vi "Get Text Label Decs from VI__ogtk.vi"(8 "error in (no error)":errorcluster, 11 "VI Refnum":refnum<vi>) -> (0 "error out":errorcluster, 2 "FP Floating Text Labels":refnum<vi>[](array[refnum]), 3 "dup VI Refnum":refnum<vi>)   [LabVIEW 2016]
doc: "Returns references to the free labels (floating text) on a VI's Front Panel."
panel:
  # "Get Text Label Decs from VI.vi\n\nReturns references to the free labels (floating text) on a VI's Front Panel.\n\nPlease visit http://www.OpenG.org to learn about the\nOpen Source LabVIEW software movement.\n\nNOTICE -- YOU MUST LEAVE THIS NOTICE IN PLACE.  PER THE TERMS OF THE LICENSE BELOW, YOU MAY SUBLICENSE THIS SOFTWARE \nIN ANY WAY THAT DOES NOT CONFLICT WITH THIS LICENSE.\n\n### BSD License (http://www.opensource.org/licenses/bsd-license.php) Begin ###\n \nCopyright (c) 2002, Jean-Pierre Drolet <drolet_jp@hotmail.com>\nCopyright (c) 2002, Jim Kring <jim@jimkring.com>\n\nAll rights reserved.\n\nRedistribution and use in source and binary forms, with or without modification, are permitted provided that the following conditions are met:\n\n    * Redistributions of source code must retain the above copyright notice, this list of conditions and the following disclaimer.\n    * Redistributions in binary form must reproduce the above copyright notice, this list of conditions and the following disclaimer in the \n       documentation and/or other materials provided with the distribution.\n    * Neither the name of SciWare, James Kring, Inc., nor the names of its contributors may be used to endorse or promote products derived \n       from this software without specific prior written permission.\n\nTHIS SOFTWARE IS PROVIDED BY THE COPYRIGHT HOLDERS AND CONTRIBUTORS \"AS IS\" AND ANY EXPRESS OR IMPLIED WARRANTIES, \nINCLUDING, BUT NOT LIMITED TO, THE IMPLIED WARRANTIES OF MERCHANTABILITY AND FITNESS FOR A PARTICULAR PURPOSE ARE \nDISCLAIMED. IN NO EVENT SHALL THE COPYRIGHT OWNER OR CONTRIBUTORS BE LIABLE FOR ANY DIRECT, INDIRECT, INCIDENTAL,\n SPECIAL, EXEMPLARY, OR CONSEQUENTIAL DAMAGES (INCLUDING, BUT NOT LIMITED TO, PROCUREMENT OF SUBSTITUTE GOODS OR \nSERVICES; LOSS OF USE, DATA, OR PROFITS; OR BUSINESS INTERRUPTION) HOWEVER CAUSED AND ON ANY THEORY OF LIABILITY, \nWHETHER IN CONTRACT, STRICT LIABILITY, OR TORT (INCLUDING NEGLIGENCE OR OTHERWISE) ARISING IN ANY WAY OUT OF THE USE \nOF THIS SOFTWARE, EVEN IF ADVISED OF THE POSSIBILITY OF SUCH DAMAGE.\n\n### BSD License End ###"
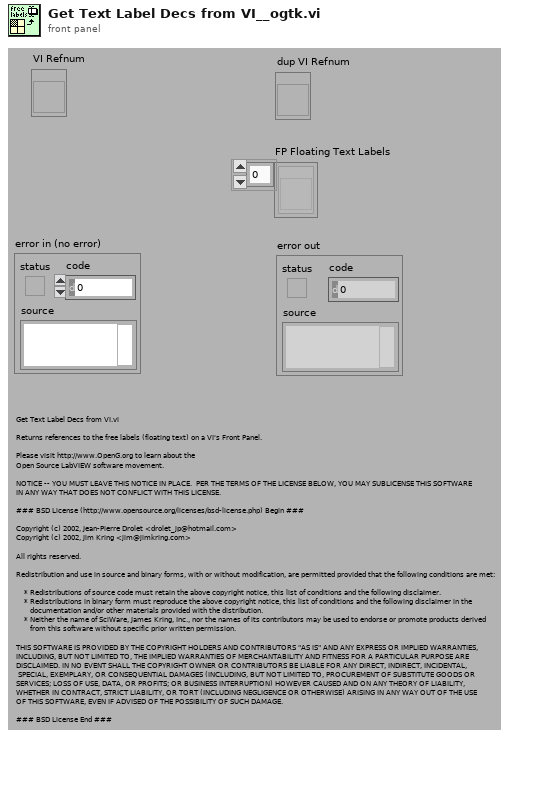
[diagram p1: front panel]
types:
  T1 = enum32{"0 <undefined>", "1 <undefined>", "2 <undefined>", "Generic", "Decoration", "Text", "Control", "ColorBox", "Boolean", "RefNum", "Variant", "Path", "ListBox", "Table", "Array", "Picture", "ActiveXContainer", "Numeric", "Digital", "NamedNumeric", "ColorRamp", "Slide", "GraphOrChart", "WaveformChart", "WaveformGraph", "IntensityChart", "IntensityGraph", "String", "IOName", "ComboBox", "Cluster", "Panel", "Knob", "NumWithScale", "Ring", "Enum", "GObject", "Plot", "Cursor", "NumericText", "Scale", "ColorScale", "GraphScale", "ColorGraphScale", "TypedRefNum", "OldKnobScale", "MCListbox", "MeasureData", "BVTag", "DAQName", "VISAName", "IVIName", "SlideScale", "TabControl", "Page", "TabArrayTabControl", "ConPane"}
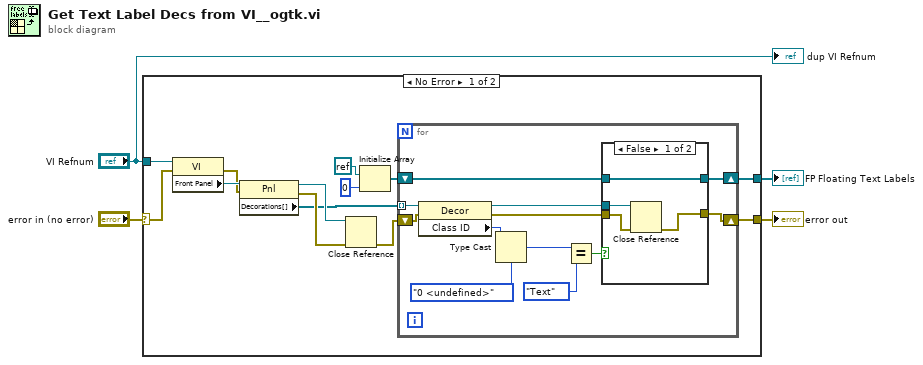
[diagram p0: block diagram]
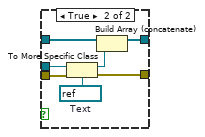
[diagram p2: hidden frame]
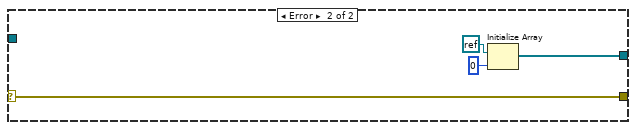
[diagram p3: hidden frame]
diagram:
  n1 = case shown="No Error" "error in (no error)" {
    selector: "error in (no error)" -> [w5 w41]
    tunnel: "VI Refnum" -> [w7 _]
    tunnel: [w15 w42] -> w4
    tunnel: [w6 w41] -> w1
    frame No Error {
      n2 = property class="VI"(reference=w7, error in=w5) -> (error out=w16:errorcluster, "Front Panel"=w17:refnum<vi>)  [unwired: 1 out]
      n3 = property class="Pnl"(reference=w17, error in=w16) -> (reference out=w10:refnum<vi>, error out=w9:errorcluster, "Decorations[]"=w8:refnum<vi>[])
      n4 = Close Reference(reference=w10, error in (no error)=w9) -> (error out=w14:errorcluster)
      n5 = Initialize Array(refnum<k0> refnum, 0 ("Dimension Size")) -> (w11:refnum<k0>[])
      n6 = for {
        tunnel: w8 -> [w29] mode=indexing
        shift-right: [w24] -> w15
        shift-left: w11 -> [w25]
        shift-right: [w18] -> w6
        shift-left: w14 -> [w20]
        n7 = property class="Decor"(reference=w29, error in=w20) -> (reference out=w23:refnum<vi>, error out=w19:errorcluster, "Class ID"=w28:u32)
        n8 = Type Cast(type=T1."0 <undefined>" ("ClassID Name"), x=w28) -> (*(type *) &x=w22:T1)
        n9 = Equal?(x=w22, y=T1."Text" ("ClassID Name")) -> (x = y?=w26:bool)
        n10 = case shown="False" w26 {
          tunnel: w25 -> [w32 w40]
          tunnel: [w32 w39] -> w24
          tunnel: w23 -> [w33 w38]
          tunnel: w19 -> [w31 w35]
          tunnel: [w30 w34] -> w18
          frame False {
            n11 = Close Reference(reference=w33, error in (no error)=w31) -> (error out=w30:errorcluster)
          }
          frame True {
            w37 = refnum<vi> refnum  # Text
            n12 = To More Specific Class(target class=w37, reference=w38, error in=w35) -> (specific class reference=w36:refnum<vi>, error out=w34:errorcluster)
            n13 = Build Array (concatenate)(w40, w36) -> (w39:refnum<vi>[])
          }
        }
      }
    }
    frame Error {
      n14 = Initialize Array(refnum<k0> refnum, 0 ("Dimension Size")) -> (w42:refnum<k0>[])
    }
  }
  "FP Floating Text Labels" <- w4
  "error out" <- w1
  "dup VI Refnum" <- "VI Refnum"
